vi "PicoScope6000Settings.vi"(0 "PS6407?":bool, 4 "Channel D Settings":T1={"Enabled"=FALSE, "Coupling"=1, "Range"=6, "Analogue Offset"=0.0, "Bandwidth"=0} {"Bandwidth" items=["Full", "20 MHz"]; "Range" items=["10 mV", "20 mV", "50 mV", "100 mV", "200 mV", "500 mV", "1 V", "2 V", "5 V", "10 V", "20 V", "50 V ", "100 V"]; "Coupling" items=["AC", "DC 1 MOhm", "DC 50 Ohm"]}, 5 "Channel B Settings":T1={"Enabled"=FALSE, "Coupling"=1, "Range"=6, "Analogue Offset"=0.0, "Bandwidth"=0} {"Bandwidth" items=["Full", "20 MHz"]; "Range" items=["10 mV", "20 mV", "50 mV", "100 mV", "200 mV", "500 mV", "1 V", "2 V", "5 V", "10 V", "20 V", "50 V ", "100 V"]; "Coupling" items=["AC", "DC 1 MOhm", "DC 50 Ohm"]}, 6 "Channel C Settings":T1={"Enabled"=FALSE, "Coupling"=1, "Range"=6, "Analogue Offset"=0.0, "Bandwidth"=0} {"Bandwidth" items=["Full", "20 MHz"]; "Range" items=["10 mV", "20 mV", "50 mV", "100 mV", "200 mV", "500 mV", "1 V", "2 V", "5 V", "10 V", "20 V", "50 V ", "100 V"]; "Coupling" items=["AC", "DC 1 MOhm", "DC 50 Ohm"]}, 7 "Channel A Settings":T1={"Enabled"=TRUE, "Coupling"=1, "Range"=6, "Analogue Offset"=0.0, "Bandwidth"=0} {"Bandwidth" items=["Full", "20 MHz"]; "Range" items=["10 mV", "20 mV", "50 mV", "100 mV", "200 mV", "500 mV", "1 V", "2 V", "5 V", "10 V", "20 V", "50 V ", "100 V"]; "Coupling" items=["AC", "DC 1 MOhm", "DC 50 Ohm"]}, 8 "Trigger Settings":T2={"Trigger Enabled"=FALSE, "Trigger Source"=enum."Channel A", "Trigger Threshold (16-bit counts)"=0, "Trigger Direction"=2, "Trigger Delay (samples)"=0, "Auto Trigger Time (ms)"=1000} {"Trigger Direction" items=["Rising"=2, "Falling"=3]}, 10 "handle in":i16, 11 "error in":errorcluster) -> (1 "Enabled array":i16[](array[numeric]), 2 "handle out":i16, 3 "error out":errorcluster)   [LabVIEW 2020]
doc: "This VI is used to set up the oscilloscope. The inputs are clusters for setting channel and simple trigger settings. Advanced triggers can be set up using PicoScope6000AdvancedTriggerSettings.vi"
uses:
  ps6000.dll
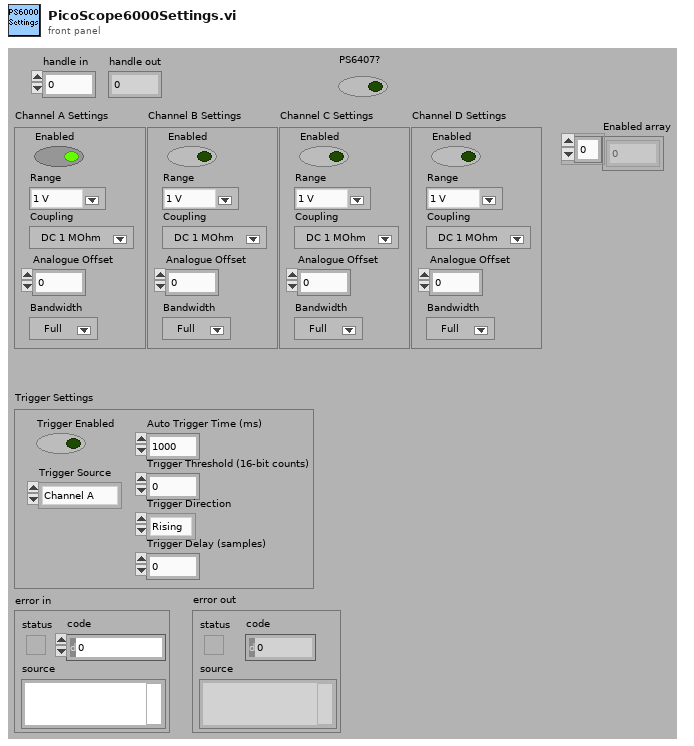
[diagram p1: front panel]
types:
  T1 = cluster{"Enabled":bool, "Coupling":u32, "Range":u32, "Analogue Offset":sgl, "Bandwidth":u32}
  T2 = cluster{"Trigger Enabled":bool, "Trigger Source":enum32{"Channel A", "Channel B", "Channel C", "Channel D", "External", "Aux."}, "Trigger Threshold (16-bit counts)":i16, "Trigger Direction":u16, "Trigger Delay (samples)":u32, "Auto Trigger Time (ms)":i16}
  T3 = cluster{"Enabled":bool, "Coupling":i32, "Range":u16, "Analogue Offset":sgl, "Bandwidth":i32}
  T4 = enum32{"Channel A", "Channel B", "Channel C", "Channel D", "External", "Aux."}
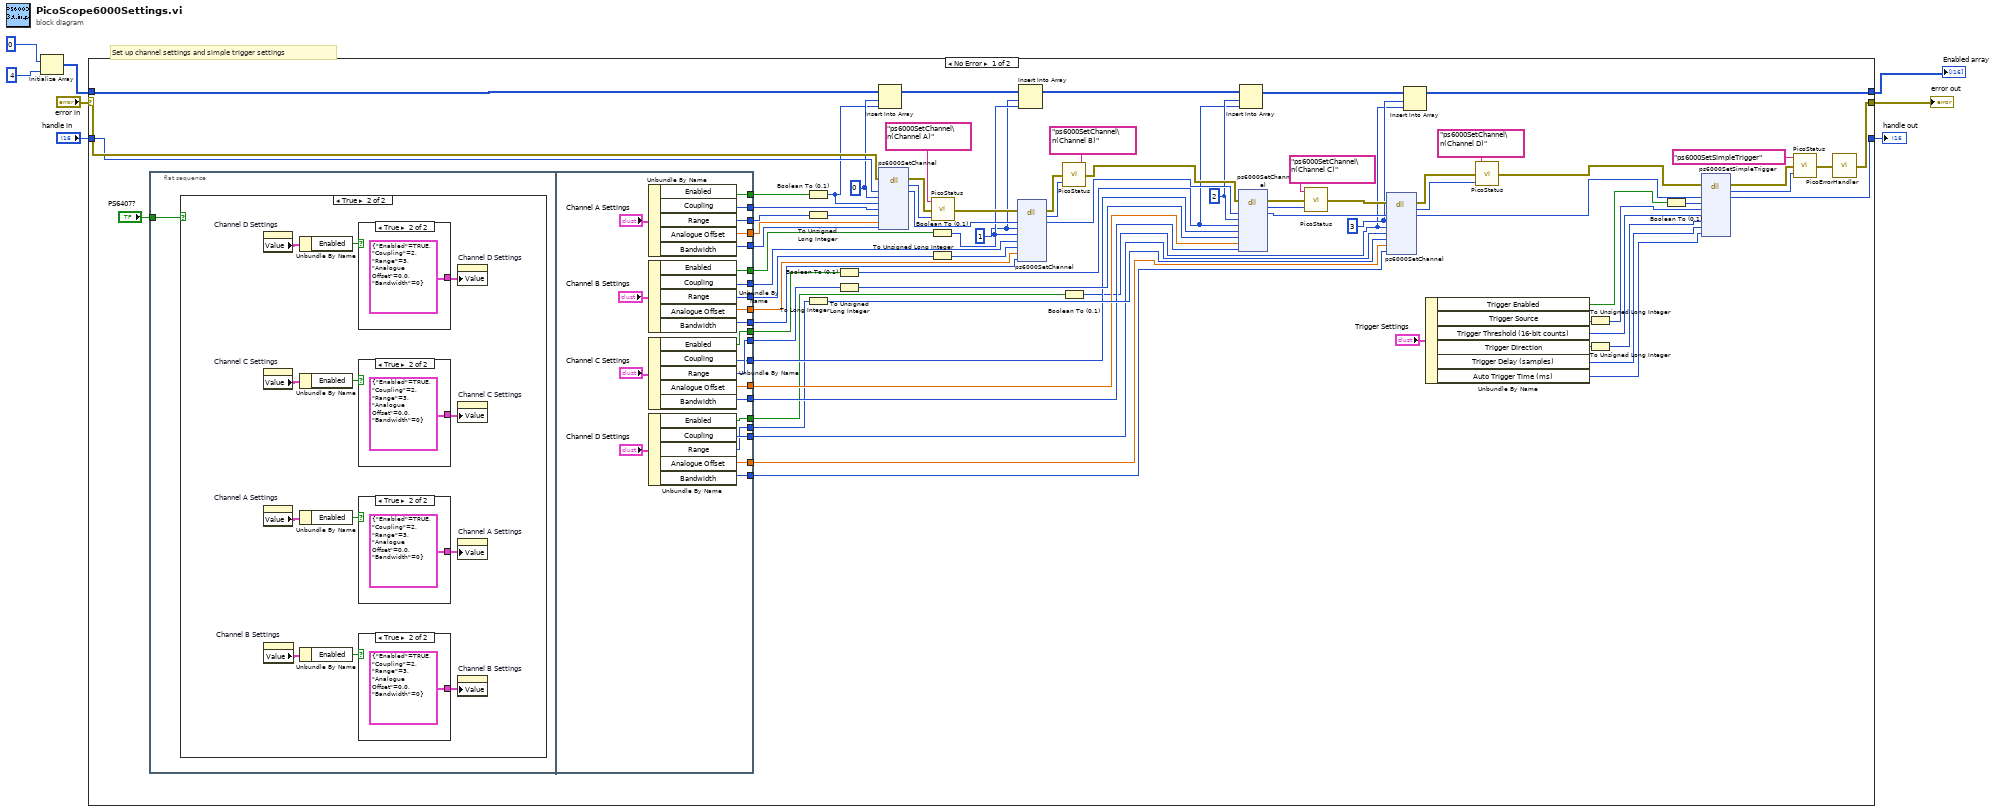
[diagram p0: block diagram]
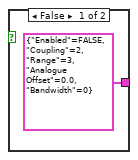
[diagram p3: hidden frame]
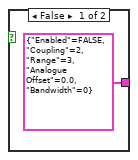
[diagram p4: hidden frame]
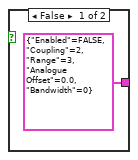
[diagram p5: hidden frame]
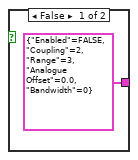
[diagram p6: hidden frame]
diagram:
  # "Set up channel settings and simple trigger settings"
  n1 = Initialize Array(i16 0, 4 ("dimension size")) -> (w3:i16[])
  n2 = case shown="No Error" "error in" {
    selector: "error in" -> [w74 w132]
    tunnel: "handle in" -> [w73 w131]
    tunnel: [w35 w131] -> w6
    tunnel: [w72 w132] -> w5
    tunnel: w3 -> [w22 w130]
    tunnel: [w9 w130] -> w1
    frame No Error {
      w11 = u32 3 ("channel")
      w13 = u32 2 ("channel")
      w16 = u32 1 ("channel")
      w21 = u32 0 ("channel")
      n3 = flat-sequence {
        tunnel: "PS6407?" -> [w85]
        tunnel: [w125] -> w65
        tunnel: [w124] -> w64
        tunnel: [w123] -> w63
        tunnel: [w122] -> w62
        tunnel: [w121] -> w61
        tunnel: [w120] -> w60
        tunnel: [w119] -> w59
        tunnel: [w118] -> w58
        tunnel: [w117] -> w57
        tunnel: [w116] -> w56
        tunnel: [w107] -> w55
        tunnel: [w115] -> w54
        tunnel: [w114] -> w53
        tunnel: [w113] -> w52
        tunnel: [w112] -> w51
        tunnel: [w111] -> w50
        tunnel: [w110] -> w49
        tunnel: [w109] -> w48
        tunnel: [w108] -> w47
        tunnel: [w106] -> w46
        frame #0 {
          n4 = case shown="True" w85 {
            frame False {
            }
            frame True {
              n5 = property on="Channel D Settings" class="Clust (strict)"() -> ("Value"=w87:T1)  [unwired: 2 in, 2 out]
              n6 = property on="Channel C Settings" class="Clust (strict)"() -> ("Value"=w89:T1)  [unwired: 2 in, 2 out]
              n7 = property on="Channel A Settings" class="Clust (strict)"() -> ("Value"=w94:T1)  [unwired: 2 in, 2 out]
              n8 = property on="Channel B Settings" class="Clust (strict)"() -> ("Value"=w92:T1)  [unwired: 2 in, 2 out]
              n9 = Unbundle By Name(w87) -> ("Enabled"=w96:bool)
              n10 = Unbundle By Name(w89) -> ("Enabled"=w97:bool)
              n11 = Unbundle By Name(w94) -> ("Enabled"=w95:bool)
              n12 = Unbundle By Name(w92) -> ("Enabled"=w91:bool)
              n13 = case shown="True" w96 {
                tunnel: [T3 {"Enabled"=FALSE, "Coupling"=2, "Range"=3, "Analogue Offset"=0.0, "Bandwidth"=0} ("Channel A Settings") T3 {"Enabled"=TRUE, "Coupling"=2, "Range"=3, "Analogue Offset"=0.0, "Bandwidth"=0} ("Channel A Settings")] -> w86
                frame False {
                }
                frame True {
                }
              }
              n14 = case shown="True" w97 {
                tunnel: [T3 {"Enabled"=FALSE, "Coupling"=2, "Range"=3, "Analogue Offset"=0.0, "Bandwidth"=0} ("Channel A Settings") T3 {"Enabled"=TRUE, "Coupling"=2, "Range"=3, "Analogue Offset"=0.0, "Bandwidth"=0} ("Channel A Settings")] -> w88
                frame False {
                }
                frame True {
                }
              }
              n15 = case shown="True" w95 {
                tunnel: [T3 {"Enabled"=FALSE, "Coupling"=2, "Range"=3, "Analogue Offset"=0.0, "Bandwidth"=0} ("Channel A Settings") T3 {"Enabled"=TRUE, "Coupling"=2, "Range"=3, "Analogue Offset"=0.0, "Bandwidth"=0} ("Channel A Settings")] -> w93
                frame False {
                }
                frame True {
                }
              }
              n16 = case shown="True" w91 {
                tunnel: [T3 {"Enabled"=FALSE, "Coupling"=2, "Range"=3, "Analogue Offset"=0.0, "Bandwidth"=0} ("Channel A Settings") T3 {"Enabled"=TRUE, "Coupling"=2, "Range"=3, "Analogue Offset"=0.0, "Bandwidth"=0} ("Channel A Settings")] -> w90
                frame False {
                }
                frame True {
                }
              }
              n17 = property on="Channel D Settings" class="Clust (strict)"("Value"=w86) -> ()  [unwired: 2 in, 2 out]
              n18 = property on="Channel C Settings" class="Clust (strict)"("Value"=w88) -> ()  [unwired: 2 in, 2 out]
              n19 = property on="Channel A Settings" class="Clust (strict)"("Value"=w93) -> ()  [unwired: 2 in, 2 out]
              n20 = property on="Channel B Settings" class="Clust (strict)"("Value"=w90) -> ()  [unwired: 2 in, 2 out]
            }
          }
        }
        frame #1 {
          n21 = Unbundle By Name("Channel A Settings") -> ("Enabled"=w125:bool, "Coupling"=w124:u32, "Range"=w123:u32, "Analogue Offset"=w122:sgl, "Bandwidth"=w121:u32)
          n22 = Unbundle By Name("Channel B Settings") -> ("Enabled"=w106:bool, "Coupling"=w120:u32, "Range"=w119:u32, "Analogue Offset"=w118:sgl, "Bandwidth"=w117:u32)
          n23 = Unbundle By Name("Channel C Settings") -> ("Enabled"=w116:bool, "Coupling"=w107:u32, "Range"=w115:u32, "Analogue Offset"=w114:sgl, "Bandwidth"=w113:u32)
          n24 = Unbundle By Name("Channel D Settings") -> ("Enabled"=w112:bool, "Coupling"=w111:u32, "Range"=w110:u32, "Analogue Offset"=w109:sgl, "Bandwidth"=w108:u32)
        }
      }
      n25 = Boolean To (0,1)(Boolean=w65) -> (0, 1=w20:i16)
      n26 = To Unsigned Long Integer(number=w63) -> (unsigned 32bit integer=w67:u32)
      n27 = To Long Integer(number=w49) -> (32bit integer=w83:i32)
      n28 = Boolean To (0,1)(Boolean=w56) -> (0, 1=w12:i16)
      n29 = To Unsigned Long Integer(number=w54) -> (unsigned 32bit integer=w84:u32)
      n30 = Insert Into Array(array=w22, index=w21, new element=w20) -> (w19:i16[])
      n31 = dll-call lib="PS6000.dll" fn="ps6000SetChannel" ("ps3000.dll:_ps3000_open_unit@0")(error in=w74, "handle"=w73, "channel"=w21, "enabled"=w20, "type"=w64, "range"=w67, "analogueOffset"=w62, "bandwidth"=w61) -> (error out=w78:errorcluster, "PICO_STATUS"=w79:u32, "handle"=w18:i16)  [unwired: 8 in, 1 out]
      n32 = Boolean To (0,1)(Boolean=w46) -> (0, 1=w17:i16)
      n33 = To Unsigned Long Integer(number=w59) -> (unsigned 32bit integer=w66:u32)
      n34 = call "PicoStatus.vi"("PICO STATUS"=w79, "error in"=w78, "source"="ps6000SetChannel\n(Channel A)") -> ("error out"=w69:errorcluster)
      n35 = dll-call lib="PS6000.dll" fn="ps6000SetChannel" ("ps3000.dll:_ps3000_open_unit@0")(error in=w69, "handle"=w18, "channel"=w16, "enabled"=w17, "type"=w60, "range"=w66, "analogueOffset"=w58, "bandwidth"=w57) -> (error out=w71:errorcluster, "PICO_STATUS"=w70:u32, "handle"=w68:i16)  [unwired: 8 in, 1 out]
      n36 = Insert Into Array(array=w19, index=w16, new element=w17) -> (w15:i16[])
      n37 = call "PicoStatus.vi"("PICO STATUS"=w70, "error in"=w71, "source"="ps6000SetChannel\n(Channel B)") -> ("error out"=w75:errorcluster)
      n38 = Boolean To (0,1)(Boolean=w51) -> (0, 1=w10:i16)
      n39 = dll-call lib="PS6000.dll" fn="ps6000SetChannel" ("ps3000.dll:_ps3000_open_unit@0")(error in=w75, "handle"=w68, "channel"=w13, "enabled"=w12, "type"=w55, "range"=w84, "analogueOffset"=w53, "bandwidth"=w52) -> (error out=w28:errorcluster, "PICO_STATUS"=w27:u32, "handle"=w24:i16)  [unwired: 8 in, 1 out]
      n40 = Insert Into Array(array=w15, index=w13, new element=w12) -> (w14:i16[])
      n41 = call "PicoStatus.vi"("PICO STATUS"=w27, "error in"=w28, "source"="ps6000SetChannel\n(Channel C)") -> ("error out"=w23:errorcluster)
      n42 = dll-call lib="PS6000.dll" fn="ps6000SetChannel" ("ps3000.dll:_ps3000_open_unit@0")(error in=w23, "handle"=w24, "channel"=w11, "enabled"=w10, "type"=w50, "range"=w83, "analogueOffset"=w48, "bandwidth"=w47) -> (error out=w26:errorcluster, "PICO_STATUS"=w25:u32, "handle"=w42:i16)  [unwired: 8 in, 1 out]
      n43 = Insert Into Array(array=w14, index=w11, new element=w10) -> (w9:i16[])
      n44 = Unbundle By Name("Trigger Settings") -> ("Trigger Enabled"=w44:bool, "Trigger Source"=w80:T4, "Trigger Threshold (16-bit counts)"=w40:i16, "Trigger Direction"=w81:u16, "Trigger Delay (samples)"=w38:u32, "Auto Trigger Time (ms)"=w37:i16)
      n45 = call "PicoStatus.vi"("PICO STATUS"=w25, "error in"=w26, "source"="ps6000SetChannel\n(Channel D)") -> ("error out"=w43:errorcluster)
      n46 = To Unsigned Long Integer(number=w80) -> (unsigned 32bit integer=w41:u32)
      n47 = To Unsigned Long Integer(number=w81) -> (unsigned 32bit integer=w39:u32)
      n48 = Boolean To (0,1)(Boolean=w44) -> (0, 1=w34:i16)
      n49 = dll-call lib="PS6000.dll" fn="ps6000SetSimpleTrigger" ("ps3000.dll:_ps3000_open_unit@0")(error in=w43, "handle"=w42, "enabled"=w34, "source"=w41, "threshold"=w40, "direction"=w39, "delay"=w38, "autoTrigger_ms"=w37) -> (error out=w32:errorcluster, "PICO_STATUS"=w31:u32, "handle"=w35:i16)  [unwired: 8 in, 1 out]
      n50 = call "PicoStatus.vi"("PICO STATUS"=w31, "error in"=w32, "source"="ps6000SetSimpleTrigger") -> ("error out"=w36:errorcluster)
      n51 = call "PicoErrorHandler.vi"("error in"=w36) -> ("error out"=w72:errorcluster)
    }
    frame Error {
    }
  }
  "handle out" <- w6
  "error out" <- w5
  "Enabled array" <- w1
